vi "solar Msg EnQ (Main).vi"(4 "DATA Array":variant[](array[variant]), 6 "MSG Array":string[](array[string]), 7 "Priority (Normal)":enum8{"Normal", "Priority", "IgnoreIfExists"}(ring), 8 "error in (no error)":errorcluster, 9 "DATA (last)":variant, 10 "MSG (last)":string, 11 "solar in":refnum<class "solar.lvclass">) -> (0 "error out":errorcluster, 1 "Timed Out?":bool, 3 "solar out":refnum<class "solar.lvclass">)   [LabVIEW 2018]
doc: "This enqueues a message to the main targets queue."
uses:
  solar.lvclass
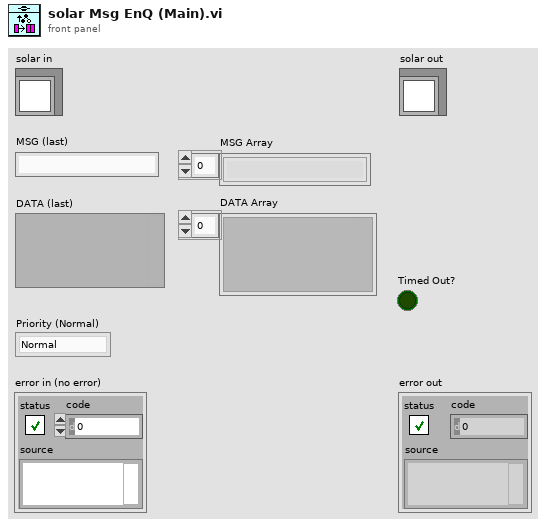
[diagram p1: front panel]
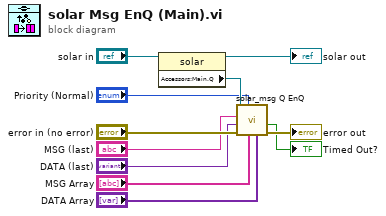
[diagram p0: block diagram]
diagram:
  n1 = property class="solar"(reference="solar in") -> (reference out=→"solar out":refnum<class "solar.lvclass">, "Accessors:Main.Q"=w9:refnum<queue>)  [unwired: 1 in, 1 out]
  n2 = call "solar_msg Q EnQ.vi"("CMD_DATA Array"="DATA Array", "CMD Array"="MSG Array", "Priority (Normal)"="Priority (Normal)", "error in (no error)"="error in (no error)", "CMD_DATA (Last)"="DATA (last)", "CMD (Last)"="MSG (last)", "Queue in"=w9) -> ("error out"=→"error out":errorcluster, "Timed Out?"=→"Timed Out?":bool)  [unwired: 2 in, 1 out]
